vi "setUp.vi"(8 "error in (no error)":errorcluster, 11 "ViewThisComponent in":refnum<class "ViewThisComponent.lvclass">) -> (0 "error out":errorcluster, 3 "ViewThisComponent out":refnum<class "ViewThisComponent.lvclass">)   [LabVIEW 2016, in "ViewThisComponent.lvclass"]
uses:
  ViewThisComponent.lvclass
  home/harini/tcs/ts_sedspectrometer/ComponentTemplateCore/ComponentModel/ComponentModel/View/View.lvclass
  ComponentTemplateCore/ComponentModel/ComponentModel/View/View.lvclass/View.ctl
  PubSubDataEvent/PubSubDataEvent.lvclass
  MiddlewareSALThisComponent/MiddlewareSALThisComponent.lvclass
  home/harini/tcs/ts_sedspectrometer/ComponentTemplateCore/ComponentModel/ComponentModel/Middleware/Middleware.lvclass
  ViewThisComponent.lvclass/ViewThisComponent.ctl
  ComponentTemplateCore/ComponentModel/ComponentModel/View/View.lvclass
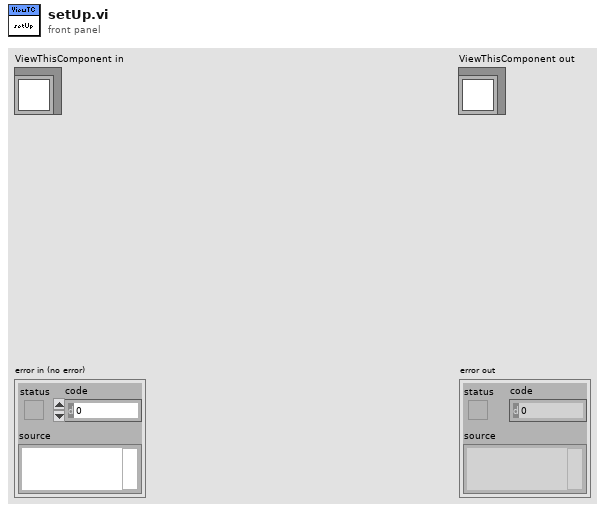
[diagram p1: front panel]
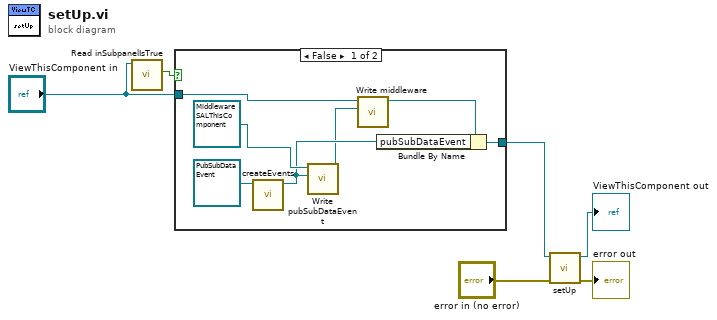
[diagram p0: block diagram]
diagram:
  n1 = call "Read inSubpanelIsTrue.vi"("View in"="ViewThisComponent in") -> ("inSubpanelIsTrue"=w1:bool)  [unwired: 9 in, 1 out]
  n2 = case shown="False" w1 {
    tunnel: "ViewThisComponent in" -> [w12 w14]
    tunnel: [w10 w14] -> w3
    frame False {
      n3 = call "createEvents.vi"("PubSubDataEvent in"=refnum<class "PubSubDataEvent.lvclass"> refnum ("PubSubDataEvent.lvclass")) -> ("PubSubDataEvent out"=w8:refnum<class "PubSubDataEvent.lvclass">)  [unwired: 9 in, 1 out]
      n4 = call "Write pubSubDataEvent.vi"("pubSubDataEvent"=w8, "MiddlewareSALThisComponent.lvclass in"=refnum<class "MiddlewareSALThisComponent.lvclass"> refnum ("MiddlewareSALThisComponent.lvclass")) -> ("MiddlewareSALThisComponent.lvclass out"=w7:refnum<class "MiddlewareSALThisComponent.lvclass">)  [unwired: 9 in]
      n5 = call "Write middleware.vi"("middleware"=w7, "View in"=w12) -> ("View out"=w11:refnum<class "ViewThisComponent.lvclass">)  [unwired: 9 in]
      n6 = Bundle By Name(cluster=w11, "pubSubDataEvent"=w8) -> (w10:refnum<class "ViewThisComponent.lvclass">)
    }
    frame True {
    }
  }
  n7 = call-parent "setUp.vi"("error in (no error)"="error in (no error)", "View in"=w3) -> ("error out"=→"error out":errorcluster, "View out"=→"ViewThisComponent out":refnum<class "ViewThisComponent.lvclass">)  [unwired: 8 in]
